vi "Read data.vi"(8 "error in (no error)":errorcluster, 11 "Node in":refnum<class "ListNode.lvclass">) -> (0 "error out":errorcluster, 2 "data":refnum<class>, 3 "Node out":refnum<class "ListNode.lvclass">)   [LabVIEW 2010, in "ListNode.lvclass"]
uses:
  ListNode.lvclass
  ListNode.lvclass/ListNode.ctl
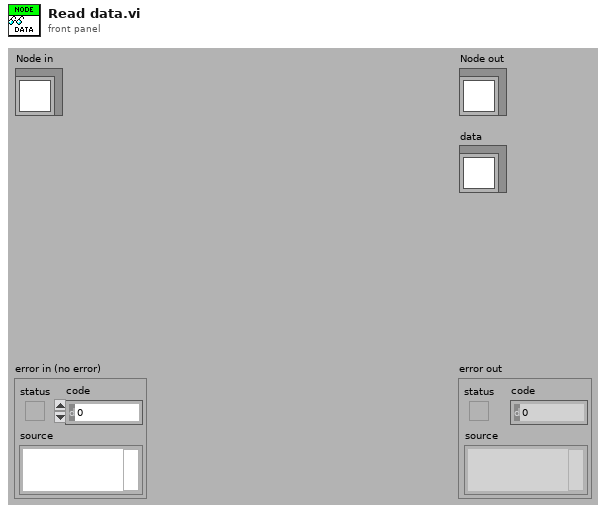
[diagram p1: front panel]
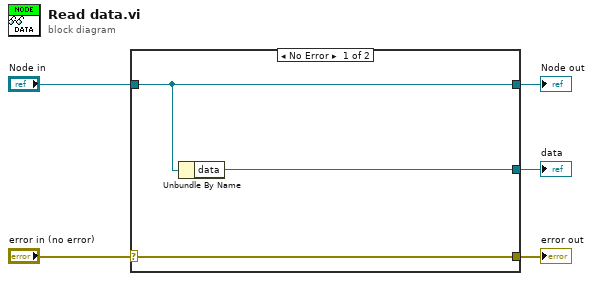
[diagram p0: block diagram]
diagram:
  n1 = case shown="No Error" "error in (no error)" {
    selector: "error in (no error)" -> [w8 w9]
    tunnel: [w8 w9] -> w4
    tunnel: [w7 w10] -> w2
    tunnel: "Node in" -> [w7 w10]
    tunnel: [w6 _] -> w1
    frame No Error {
      n2 = Unbundle By Name(w7) -> ("data"=w6:refnum<class>)
    }
    frame Error {
    }
  }
  "error out" <- w4
  "Node out" <- w2
  "data" <- w1
